vi "checkTurnState.vi"(9 "Robot":refnum<class "Robot.lvclass">, 10 "Game":refnum<class "Game.lvclass">) -> (3 "robotKickState":T1)   [LabVIEW 2020, in "KickToSkill.lvclass"]
uses:
  KickToSkill.lvclass
  Robot_class/robotKickToStates.ctl
  Robot_class/Robot.lvclass
  Game_class/Game.lvclass
  Robot_class/Robot.lvclass/Robot.ctl
  Game_class/Game.lvclass/Game.ctl
  Parameters_class/Parameters.lvclass/Parameters.ctl
  Ball_class/Ball.lvclass/Ball.ctl
  RobotFeedback/RobotFeedback.lvclass/RobotFeedback.ctl
  RobotFeedback/Read dribblerContactToBall.vi
  Game_class/Read Parameters.lvclass.vi
  Game_class/Read Utilities.lvclass.vi
  Game_class/Read BallRef.vi
  Game_class/Read NewParameters.vi
  Game_class/Read RobotsFeedback.vi
  Ball_class/Read Valid.vi
  Parameters_class/Read TouchDistance.vi
  Robot_class/Read id.vi
  Parameters_class/Parameters.lvclass
  Utilities_class/Utilities.lvclass
  Ball_class/Ball.lvclass
  RobotFeedback/RobotFeedback.lvclass
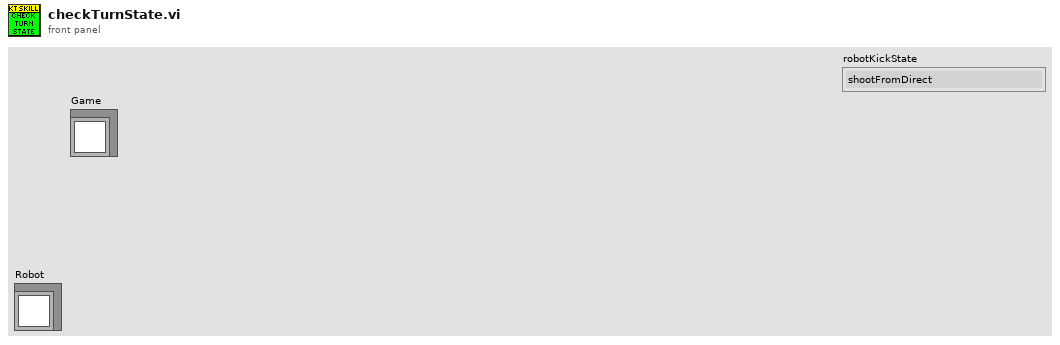
[diagram p1: front panel]
types:
  T1 = typedef "robotKickToStates.ctl" = enum16{"shootFromDirect", "avoidCollideBall", "goToBackBall", "none", "walk", "turn", "oldKickToShoot", "oldKickToGoToBackBall", "shoot"}
  T2 = typedef "NewParameters.ctl" = cluster{"PenaltyDistance":dbl, "DistanceAttackerToBackBall":dbl, "Division":enum16{"Div B", "Div A"}, "DistanceToAvoidyEnemyRobot":dbl, "BallPlacementDistance":dbl, "DisatanceBehindBallToStealBall":dbl, "MaxDistanceToPositionKickoff":dbl, "BlockEnemyTarget":bool, "MaxStopVAng":dbl, "DistanceMarkerToEnemy":dbl, "IgnoreDribblerContact":bool, "DistanceToBeginEnemyPosession":dbl, "GoToBallWhenEnemyNotMoving":bool, "EnemyDistanceToReduceVelocity":dbl, "TurnOnEnemyDistanceToReduceVelocity":bool, "EnemyDistanceToShootOutBall":dbl, "DefenseKickBall":bool, "MoreKickToGoal? (0-0.3)":dbl, "ChipKickInEnemyField":bool, "ShootOutRobotId":dbl, "FieldLenghtDenominatorInShootOut":dbl, "GoalieKickForce":dbl, "AdjustPositionInBallPlacement":bool, "PowerGodPass":dbl, "VelocityAbortEnemyPos":dbl, "MaxDistToBeginPass":dbl, "MinDistToBeginPass":dbl, "VelocityInDirects":dbl, "BadDribblerIDs":i32[], "NewKickToDistanceAroundBall":dbl, "PowerAvoidColisionMarker":dbl, "DistanceToAvoidColisionMarker":dbl, "AvoidBallKick":dbl, "DistanceTryKick":dbl, "SuicideKickDIstance":dbl, "SuicideKickAtck":bool, "SuicideAngleDistance":dbl, "SuicideKickDefense":bool, "AvoidAimLessKick":dbl, "KIckForceWithChipKick":dbl, "DistanceToAvoidyEnemyShootRobot ":dbl, "NumberOfMarkers":dbl, "PotField":bool, "PIDLateral":bool}
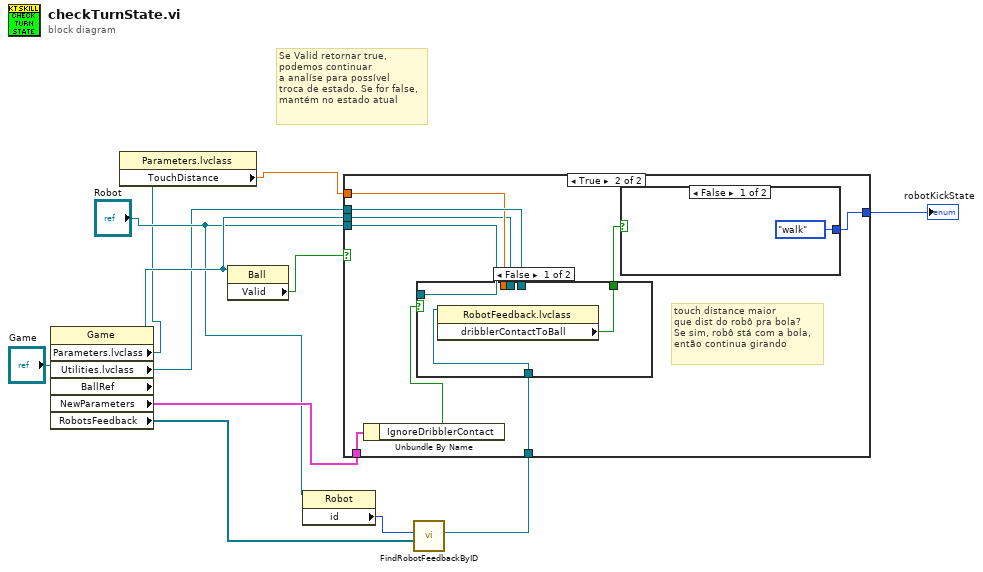
[diagram p0: block diagram]
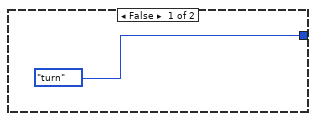
[diagram p2: hidden frame]
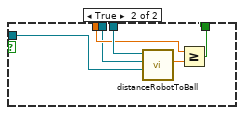
[diagram p3: hidden frame]
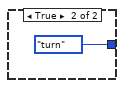
[diagram p4: hidden frame]
diagram:
  # "Se Valid retornar true,\npodemos continuar\na analíse para possível\ntroca de estado. Se for false,\nmantém no estado atual"
  n1 = property class="Game"(reference="Game") -> ("Parameters.lvclass"=w2:refnum<class "Parameters.lvclass">, "Utilities.lvclass"=w3:refnum<class "Utilities.lvclass">, "BallRef"=w9:refnum<class "Ball.lvclass">, "NewParameters"=w8:T2, "RobotsFeedback"=w7:refnum<class "RobotFeedback.lvclass">[])  [unwired: 1 in, 2 out]
  n2 = property class="Parameters.lvclass"(reference=w2) -> ("TouchDistance"=w1:dbl)  [unwired: 1 in, 2 out]
  n3 = property class="Ball"(reference=w9) -> ("Valid"=w12:bool)  [unwired: 1 in, 2 out]
  n4 = property class="Robot"(reference="Robot") -> ("id"=w5:i32)  [unwired: 1 in, 2 out]
  n5 = call "FindRobotFeedbackByID.vi"("RobotsFeedback"=w7, "id"=w5) -> ("RobotFeedback.lvclass"=w4:refnum<class "RobotFeedback.lvclass">)  [unwired: 6 in, 3 out]
  n6 = case shown="True" w12 {
    tunnel: w3 -> [_ w22]
    tunnel: "Robot" -> [_ w21]
    tunnel: w1 -> [_ w20]
    tunnel: [robotKickToStates."turn" ("robotKickState") w19] -> w11
    tunnel: w9 -> [_ w18]
    tunnel: w8 -> [_ w16]
    tunnel: w4 -> [_ w14]
    frame False {
    }
    frame True {
      # "touch distance maior\nque dist do robô pra bola?\nSe sim, robô stá com a bola,\nentão continua girando"
      n7 = Unbundle By Name(w16) -> ("IgnoreDribblerContact"=w15:bool)
      n8 = case shown="False" w15 {
        tunnel: w22 -> [_ w30]
        tunnel: w21 -> [_ w29]
        tunnel: w20 -> [_ w27]
        tunnel: w18 -> [_ w26]
        tunnel: [w23 w25] -> w17
        tunnel: w14 -> [w24 _]
        frame False {
          n9 = property class="RobotFeedback.lvclass"(reference=w24) -> ("dribblerContactToBall"=w23:bool)  [unwired: 1 in, 2 out]
        }
        frame True {
          n10 = call "distanceRobotToBall.vi"("Robot"=w29, "Ball"=w26, "Utilities in"=w30) -> ("Distance Robot To Ball"=w28:dbl)  [unwired: 6 in, 2 out]
          n11 = Greater Or Equal?(x=w27, y=w28) -> (x >= y?=w25:bool)
        }
      }
      n12 = case shown="False" w17 {
        tunnel: [robotKickToStates."walk" robotKickToStates."turn" ("robotKickState")] -> w19
        frame False {
        }
        frame True {
        }
      }
    }
  }
  "robotKickState" <- w11
